vi "Scope_Data.vi"(0 "VDDA":dbl=3.3, 1 "Enum":T6(ring)=enum."I2C_SU_HD_START", 3 "Record Length":i32=2000000, 5 "error in (no error)":errorcluster) -> (12 "output cluster":T1={"Result_Name_Str1"="tSU_Data_ns", "Result_Val1"=864.0093750000001, "Result_Name_Str2"="tHD_Data_ns", "Result_Val2"=1006.8265625, "Result_P/F__Str"="PASSED", "Result_Bool"=TRUE}, 14 "SU_DATA(ns)":dbl=864.0093750000001, 15 "HD_DATA(ns)":dbl=1006.8265625, 16 "ACKs":T3={"Reg Address ACK"=TRUE, "Address ACK"=TRUE, "Data ACK"=TRUE}, 17 "Address_Data":T2={"Data"=82, "Address"=77, "Reg Address"=102} {"Data" format="%.0x"; "Address" format="%.0x"; "Reg Address" format="%.0x"}, 19 "error out":errorcluster)   [LabVIEW 2019]
uses:
  <vilib>/addons/jitter/shared/controls/ja_crossing times.ctl
  <vilib>/addons/jitter/shared/controls/ja_slope (two options).ctl
  <vilib>/addons/jitter/shared/controls/ja_state_settings.ctl
  <vilib>/addons/jitter/shared/controls/ja_reference level settings.ctl
  <userlib>/_TI-LA/Instr Drivers/Oscilloscope/MSO5X/Driver/Base/Public/Data/Low Level/Fetch (Waveform).vi
  <vilib>/addons/jitter/level/support/State Levels (DBL).vi
  <vilib>/addons/jitter/level/support/Reference Levels (waveform in, DBL).vi
  <vilib>/addons/jitter/level/support/Find Transitions (DBL).vi
  <vilib>/addons/jitter/timing/support/Level Crossing (Transitions in, DBL).vi
  <userlib>/_TI-LA/Instr Drivers/Oscilloscope/MSO5X/Driver/Base/Tektronix MSO5X Series.lvlib
  <vilib>/addons/jitter/NI_JAT.lvlib
panel:
  out "tBUF(ns)":dbl=32.37685263084059
  out "Result_Name_Str2":string="tHD_Data_ns"
  out "Result_Name_Str1":string="tSU_Data_ns"
  out "Result_Val2":dbl=1006.8265625 format="%#_13g"
  out "Result_Val1":dbl=864.0093750000001 format="%#_13g"
  out "Result_P/F__Str":string="PASSED"
  out "tHIGH(ns)":dbl=0.9820852205979463
  out "tLOW(ns)":dbl=32.37685263084059
  out "HD_START(ns) 400K":dbl=0.9820852205979463
  out "SU_START(ns) 400K":dbl=32.37685263084059
  out "SU_STOP(ns)":dbl=32.37685263084059
  in  "crossing level 2":dbl=nan
  out "error out 2":errorcluster
  out "level crossings 2":T4={"indexes"=[138886.34765625, 144273.98567708334, 150623.021484375, 168977.31901041666, 175242.021484375, 177621.478515625, 183858.04296875, 194311.65234375, 200551.01432291666, 217971.31901041666, 221517.021484375, 227093.31901041666, 233441.521484375, 251871.978515625, 258263.021484375, 260683.95703125, 266952.021484375, 277424.478515625, 283695.0143229167, 302509.95703125, 308780.521484375, 319308.478515625, 325619.521484375, 343952.978515625, 350295.0143229167, 379433.478515625], "t0"=timestamp(3.199999999681756e-10 s since 1904-01-01), "dt"=3.2e-10, "slope"=-1, "crossing level"=1.5548437499999999} {"crossing level" format="%#_6p"; "slope" items=["Rising Edge"=1, "Falling Edge"=-1]; "dt" format="%#_6p"}
  out "waveform dup 2":waveform(dbl)={"t0"=timestamp(3.199999999681756e-10 s since 1904-01-01), "dt"=3.2e-10, "Y"=array[2000000 elements]}
  out "Clock_size":i32=62
  out "Reg Address  Binary":bool[](array[boolean])=[FALSE, TRUE, TRUE, FALSE, FALSE, TRUE, TRUE]
  out "Reg Address ACK":bool=TRUE
  out "Reg Address":u32=102 format="%.0x"
  out "Address Binary":bool[](array[boolean])=[TRUE, FALSE, TRUE, TRUE, FALSE, FALSE, TRUE]
  out "Address ACK":bool=TRUE
  out "Address":u32=77 format="%.0x"
  out "Data ACK":bool=TRUE
  out "Data":u32=82 format="%.0x"
  out "Data Binary":bool[](array[boolean])=[FALSE, TRUE, FALSE, FALSE, TRUE, FALSE, TRUE, FALSE]
  out "Ch2 Waveform Graph":waveform(dbl)(graph)={"t0"=timestamp(3.199999999681756e-10 s since 1904-01-01), "dt"=3.2e-10, "Y"=array[2000000 elements]}
  in  "Channel (CH2)":string="CH4\nCH4"
  out "waveform dup":waveform(dbl)={"t0"=timestamp(3.199999999681756e-10 s since 1904-01-01), "dt"=3.2e-10, "Y"=array[2000000 elements]}
  out "level crossings":T4={"indexes"=[134617.7548828125, 136769.490234375, 140906.7548828125, 145395.7451171875, 149365.509765625, 153842.7451171875, 157724.509765625, 161770.490234375, 165654.7548828125, 170056.490234375, 173946.2548828125, 178701.490234375, 182599.509765625, 187087.2451171875, 190983.7548828125, 195395.2451171875, 199290.7548828125, 203779.49674479166, 207673.2548828125, 211846.7451171875, 215894.2548828125, 220221.490234375, 223687.7548828125, 228251.7451171875, 232184.509765625, 236707.490234375, 240600.7548828125, 244653.7451171875, 248545.7548828125, 252990.490234375, 256888.509765625, 261725.7451171875, 265615.8365885417, 270174.2451171875, 274060.509765625, 278504.490234375, 282399.509765625, 286883.2451171875, 290775.509765625, 295023.7451171875, 299027.509765625, 303667.490234375, 307560.7548828125, 312007.7451171875, 315943.509765625, 320467.7451171875, 324324.2548828125, 328843.830078125, 332734.7548828125, 336709.490234375, 340632.509765625, 345108.7451171875, 349036.8365885417, 353441.7451171875, 357333.509765625, 361309.830078125, 365239.7548828125, 369413.490234375, 373381.7548828125, 377436.490234375, 381484.2548828125, 383687.7451171875], "t0"=timestamp(3.199999999681756e-10 s since 1904-01-01), "dt"=3.2e-10, "slope"=-1, "crossing level"=1.7388281250000002} {"crossing level" format="%#_6p"; "slope" items=["Rising Edge"=1, "Falling Edge"=-1]; "dt" format="%#_6p"}
  in  "crossing level":dbl=nan
  out "VISA resource name out":refnum<visa-resource-name>="MSO54_D03"
  out "Ch1 Waveform Graph":waveform(dbl)(graph)={"t0"=timestamp(3.199999999681756e-10 s since 1904-01-01), "dt"=3.2e-10, "Y"=array[2000000 elements]}
  in  "VISA resource name":refnum<visa-resource-name>="MSO54_D03"
  in  "Channel (CH1)":string="CH1"
  in  "Maximum Time (100000ms)":u32=100000
  in  "Starting Point (1)":i32=1
  in  "Ref Waveform Type":u16(ring) items=["Normal", "Came from a MATH"]
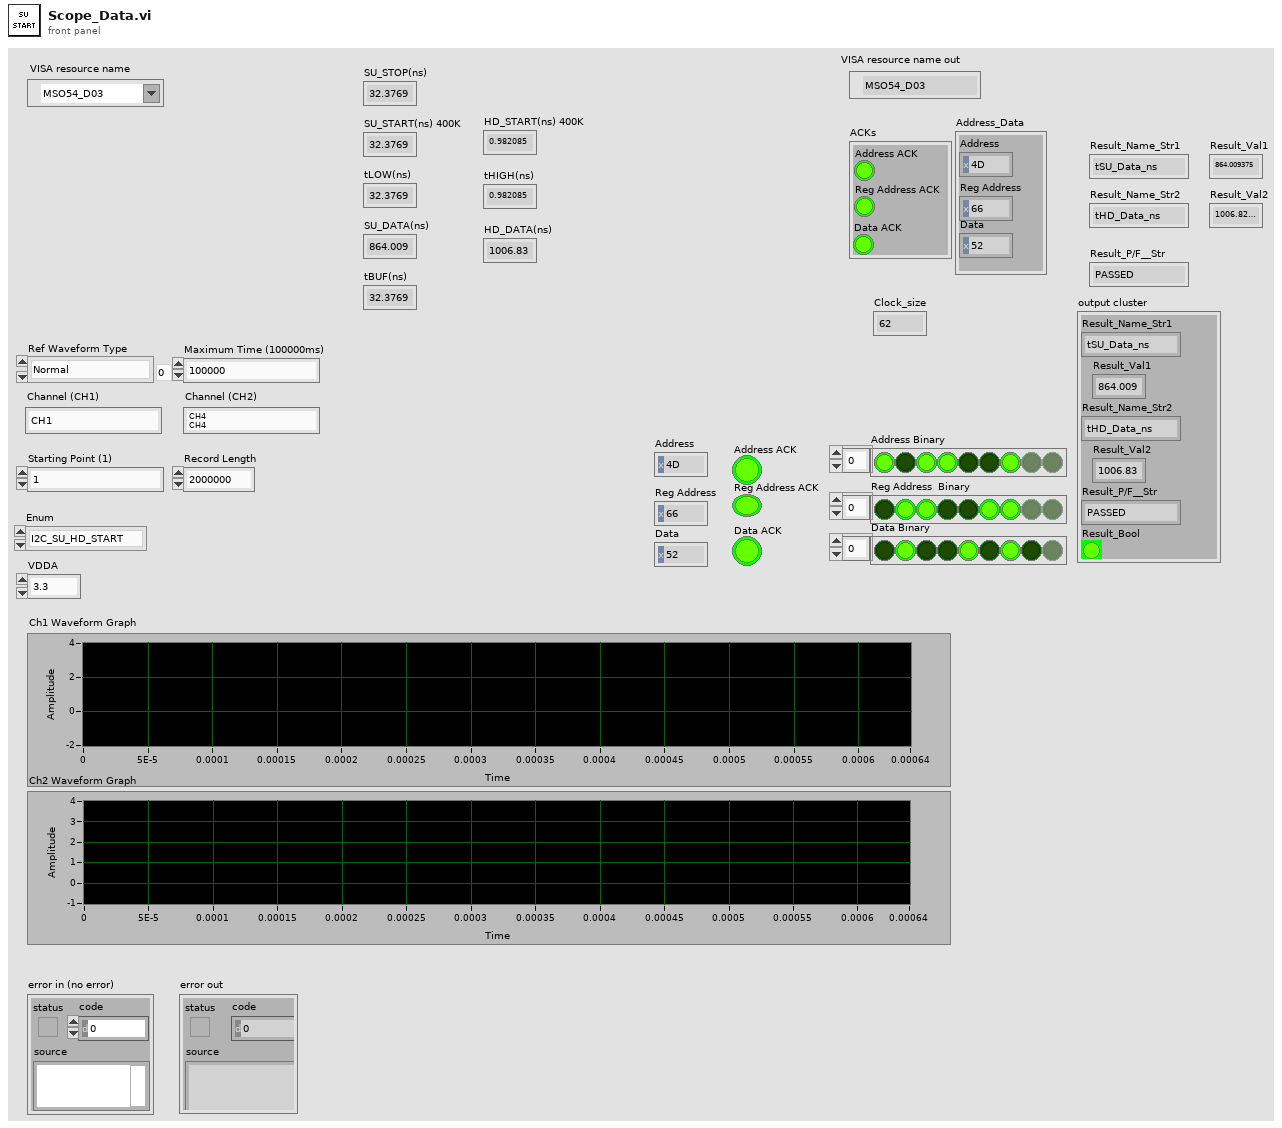
[diagram p1: front panel]
types:
  T1 = cluster{"Result_Name_Str1":string, "Result_Val1":dbl, "Result_Name_Str2":string, "Result_Val2":dbl, "Result_P/F__Str":string, "Result_Bool":bool}
  T2 = cluster{"Data":u32, "Address":u32, "Reg Address":i8}
  T3 = cluster{"Reg Address ACK":bool, "Address ACK":bool, "Data ACK":bool}
  T4 = typedef "NI_JAT.lvlib/ja_crossing times.ctl" = cluster{"indexes":dbl[], "t0":timestamp, "dt":dbl, "slope":T5, "crossing level":dbl}
  T5 = typedef "NI_JAT.lvlib/ja_slope (two options).ctl" = i16
  T6 = enum16{"I2C_Single_byte", "I2C_SU_HD_START", "I2C_SU_HD_DATA", "I2C_SU_STOP", "I2C_CLOCK_HIGH_LOW", "I2C_BUF"}
  T7 = cluster{"Data":u32, "Address":u32, "Reg Address":u32}
  T8 = typedef "NI_JAT.lvlib/ja_state_settings.ctl" = cluster{"method":enum32{"histogram", "peak", "auto select", "auto select independent"}, "histogram size":i32, "histogram method":enum16{"mode"}, "search width/total bins":dbl}
  T9 = typedef "NI_JAT.lvlib/ja_reference level settings.ctl" = cluster{"high ref level":dbl, "mid ref level":dbl, "low ref level":dbl, "ref units":u16}
  T10 = typedef "NI_JAT.lvlib/ja_state_levels.ctl" = cluster{"amplitude":dbl, "high state level":dbl, "low state level":dbl}
  T11 = typedef "NI_JAT.lvlib/ja_reference level.ctl" = cluster{"high ref level":dbl, "mid ref level":dbl, "low ref level":dbl}
  T12 = typedef "NI_JAT.lvlib/ja_transition.ctl" = cluster{"transition":T13[], "state levels":T10, "ref levels":T11}
  T13 = typedef "NI_JAT.lvlib/ja_edge.ctl" = cluster{"start index":dbl, "end index":dbl, "slope":T5}
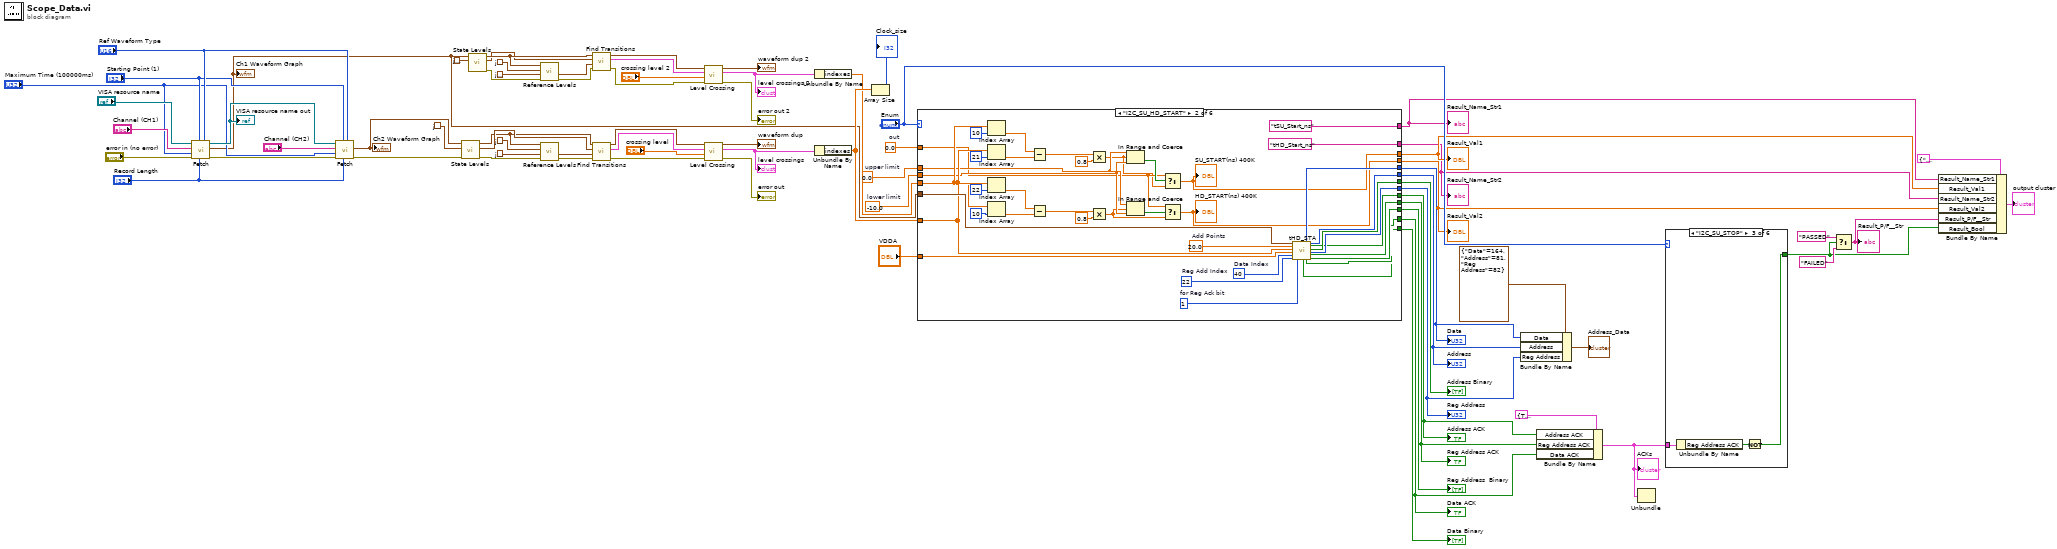
[diagram p0: block diagram]
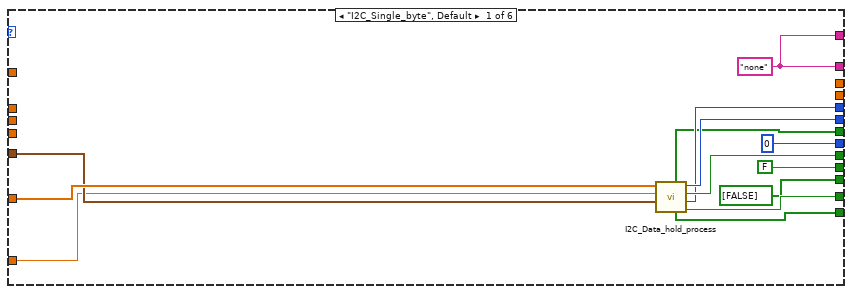
[diagram p2: hidden frame]
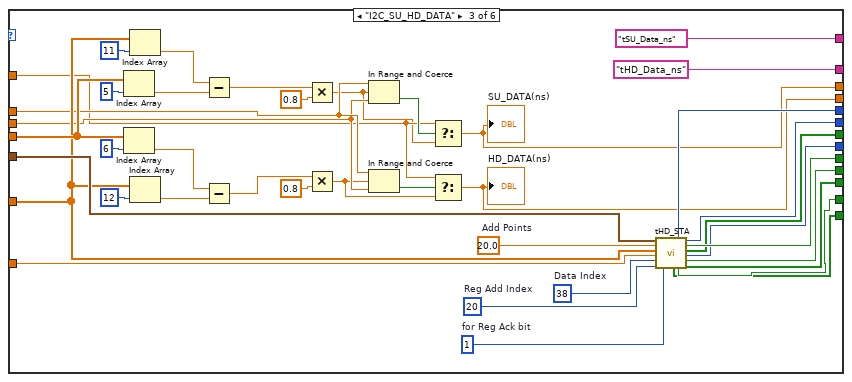
[diagram p3: hidden frame]
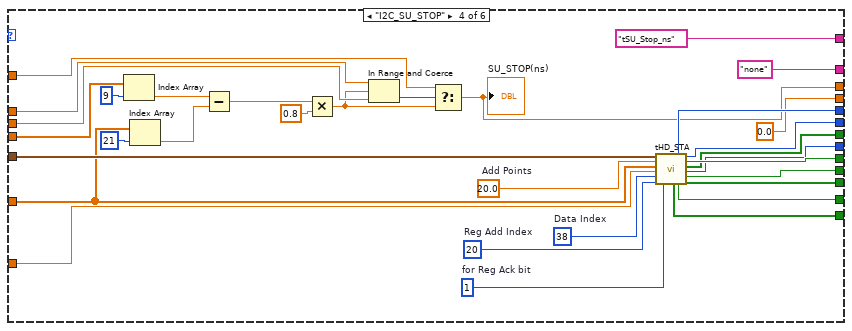
[diagram p4: hidden frame]
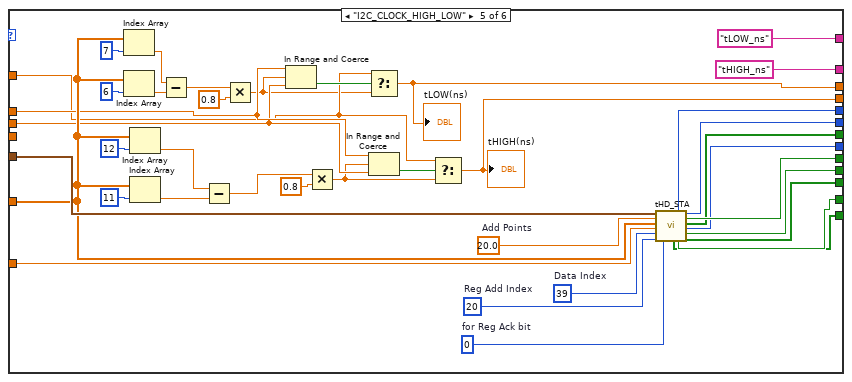
[diagram p5: hidden frame]
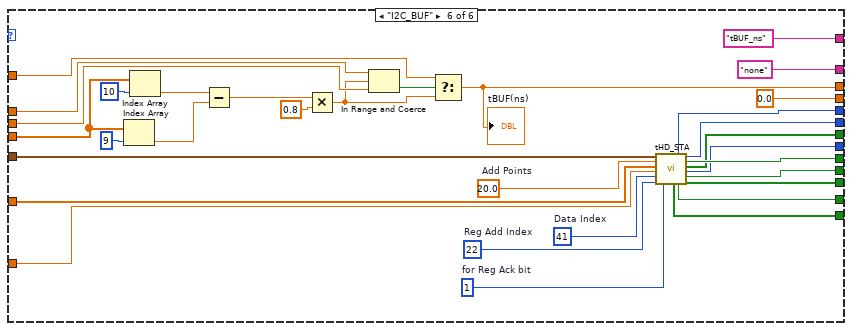
[diagram p6: hidden frame]
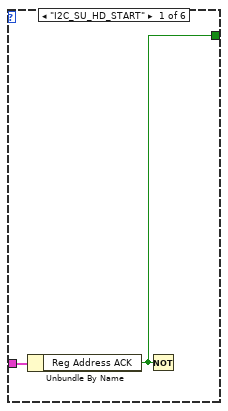
[diagram p7: hidden frame]
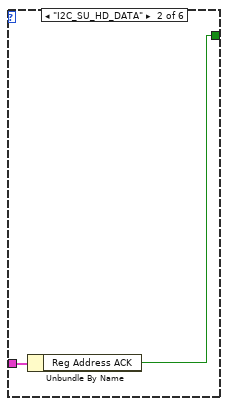
[diagram p8: hidden frame]
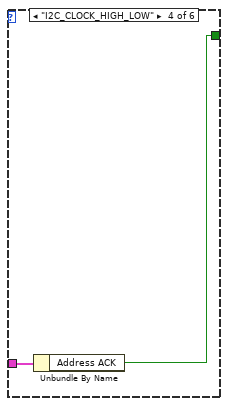
[diagram p9: hidden frame]
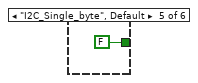
[diagram p10: hidden frame]
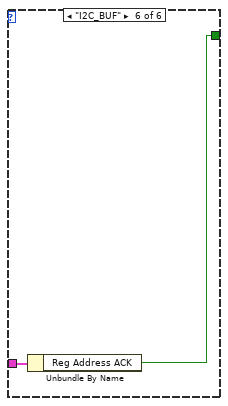
[diagram p11: hidden frame]
diagram:
  w14 = 0.0  # out
  w15 = -10.0  # lower limit
  w16 = 0.0  # upper limit
  n1 = call-poly <userlib>:"Fetch.vi"("Ref Waveform Type"="Ref Waveform Type", "Ending Point (2500)"="Record Length", "Starting Point (1)"="Starting Point (1)", "error in (no error)"="error in (no error)", "Maximum Time (100000ms)"="Maximum Time (100000ms)", "Channel (CH1)"="Channel (CH1)", "VISA resource name"="VISA resource name") -> ("error out"=w57:errorcluster, "Waveform Graph"=w29:waveform(dbl), "VISA resource name out"=w56:refnum<visa-resource-name>)  [unwired: 2 in]
  "Ch1 Waveform Graph" <- w29
  "VISA resource name out" <- w56
  n2 = call-poly <userlib>:"Fetch.vi"("Ref Waveform Type"="Ref Waveform Type", "Ending Point (2500)"="Record Length", "Starting Point (1)"="Starting Point (1)", "error in (no error)"=w57, "Maximum Time (100000ms)"="Maximum Time (100000ms)", "Channel (CH1)"="Channel (CH2)", "VISA resource name"=w56) -> ("error out"=w51:errorcluster, "Waveform Graph"=w52:waveform(dbl))  [unwired: 2 in, 1 out]
  "Ch2 Waveform Graph" <- w52
  n3 = call-poly <vilib>:"State Levels.vi"("error in"=w51, "state levels settings"=T8 {"method"=enum."histogram", "histogram size"=256, "histogram method"=enum."mode", "search width/total bins"=0.45}, "waveform"=w52) -> ("error out"=w49:errorcluster, "state levels"=w68:T10, "waveform dup"=w64:waveform(dbl))  [unwired: 6 in]
  n4 = call-poly <vilib>:"State Levels.vi"("state levels settings"=T8 {"method"=enum."histogram", "histogram size"=256, "histogram method"=enum."mode", "search width/total bins"=0.45}, "waveform"=w29) -> ("error out"=w43:errorcluster, "state levels"=w33:T10, "waveform dup"=w37:waveform(dbl))  [unwired: 7 in]
  n5 = call-poly <vilib>:"Reference Levels.vi"("error in"=w43, "reference levels settings"=T9 {"high ref level"=90.0, "mid ref level"=50.0, "low ref level"=10.0, "ref units"=1}, "state levels settings"=T8 {"method"=enum."histogram", "histogram size"=256, "histogram method"=enum."mode", "search width/total bins"=0.45} ("state levels settings 2"), "waveform"=w37) -> ("error out"=w44:errorcluster, "reference levels"=w40:T11)  [unwired: 4 in, 2 out]
  n6 = call-poly <vilib>:"Reference Levels.vi"("error in"=w49, "reference levels settings"=T9 {"high ref level"=90.0, "mid ref level"=50.0, "low ref level"=10.0, "ref units"=1}, "state levels settings"=T8 {"method"=enum."histogram", "histogram size"=256, "histogram method"=enum."mode", "search width/total bins"=0.45} ("state levels settings 2"), "waveform"=w64) -> ("error out"=w48:errorcluster, "reference levels"=w61:T11)  [unwired: 4 in, 2 out]
  n7 = call-poly <vilib>:"Find Transitions.vi"("error in (no error)"=w44, "reference levels"=w40, "state levels"=w33, "waveform"=w37) -> ("error out"=w42:errorcluster, "transitions"=w35:T12, "waveform dup"=w34:waveform(dbl))  [unwired: 5 in]
  n8 = call-poly <vilib>:"Find Transitions.vi"("error in (no error)"=w48, "reference levels"=w61, "state levels"=w68, "waveform"=w64) -> ("error out"=w50:errorcluster, "transitions"=w66:T12, "waveform dup"=w67:waveform(dbl))  [unwired: 5 in]
  n9 = call-poly <vilib>:"Level Crossing.vi"("error in (no error)"=w42, "crossing level"="crossing level 2", "transitions"=w35, "waveform"=w34) -> ("error out"=→"error out 2":errorcluster, "level crossings"=w41:T4, "waveform dup"=→"waveform dup 2":waveform(dbl))  [unwired: 5 in]
  "level crossings 2" <- w41
  n10 = call-poly <vilib>:"Level Crossing.vi"("error in (no error)"=w50, "crossing level"="crossing level", "transitions"=w66, "waveform"=w67) -> ("error out"=→"error out":errorcluster, "level crossings"=w60:T4, "waveform dup"=→"waveform dup":waveform(dbl))  [unwired: 5 in]
  "level crossings" <- w60
  n11 = Unbundle By Name(w41) -> ("indexes"=w28:dbl[])
  n12 = Unbundle By Name(w60) -> ("indexes"=w46:dbl[])
  n13 = Array Size(array=w46) -> (size(s)=→"Clock_size":i32)
  n14 = case shown="\"I2C_SU_HD_START\"" "Enum" {
    tunnel: w46 -> [w87 w108 w146 w181 w219 w263]
    tunnel: w29 -> [w86 w126 w167 w199 w238 w264]
    tunnel: "VDDA" -> [w85 w127 w166 w198 w237 w239]
    tunnel: [bool[] [FALSE] ("Reg Address  Binary") w125 w159 w189 w230 w254] -> w13
    tunnel: [FALSE ("Reg Address ACK") w124 w160 w190 w231 w255] -> w12
    tunnel: [u32 0 ("Reg Address") w123 w161 w191 w232 w257] -> w11
    tunnel: [w80 w122 w162 w192 w233 w256] -> w10
    tunnel: [w84 w121 w163 w193 w234 w258] -> w9
    tunnel: [w83 w120 w164 w194 w235 w259] -> w8
    tunnel: [w81 w119 w158 w188 w229 w253] -> w7
    tunnel: [w82 w118 w165 w195 w236 w260] -> w6
    tunnel: [w79 w117 w157 w187 w228 w252] -> w5
    tunnel: w28 -> [_ w107 w148 w182 _ w251]
    tunnel: [w75 "tSU_Start_ns" "tSU_Data_ns" "tSU_Stop_ns" "tLOW_ns" "tBUF_ns"] -> w4
    tunnel: [_ w100 w139 w175 w212 w249] -> w3
    tunnel: [w75 "tHD_Start_ns" "tHD_Data_ns" "none" "tHIGH_ns" "none"] -> w2
    tunnel: [_ w99 w140 0.0 w211 0.0] -> w1
    tunnel: w16 -> [_ w96 w136 w173 w208 w247]
    tunnel: w15 -> [_ w95 w135 w172 w207 w246]
    tunnel: w14 -> [_ w94 w134 w171 w206 w245]
    frame "I2C_Single_byte", Default {
      w75 = "none"
      n15 = call "I2C_Data_hold_process.vi"("waveform"=w86, "VDDA"=w85, "Index"=w87) -> ("Data ACK"=w81:bool, "Data"=w82:u32, "Address ACK"=w84:bool, "Address"=w83:u32, "Data Binary"=w79:bool[], "Address Binary"=w80:bool[])  [unwired: 3 in]
    }
    frame "I2C_SU_HD_START" {
      w89 = 1  # for Reg Ack bit
      w88 = 20.0  # Add Points
      w91 = 22  # Reg Add Index
      w90 = 40  # Data Index
      n16 = Index Array(array=w107, index=10) -> (element=w105:dbl)
      n17 = Index Array(array=w108, index=21) -> (element=w106:dbl)
      n18 = Index Array(array=w108, index=22) -> (element=w103:dbl)
      n19 = Index Array(array=w107, index=10) -> (element=w104:dbl)
      n20 = Subtract(x=w105, y=w106) -> (x-y=w114:dbl)
      n21 = Subtract(x=w103, y=w104) -> (x-y=w110:dbl)
      n22 = Multiply(x=w114, y=0.8) -> (x*y=w93:dbl)
      n23 = Multiply(x=w110, y=0.8) -> (x*y=w92:dbl)
      n24 = In Range and Coerce(upper limit=w96, x=w93, lower limit=w95) -> (In Range?=w98:bool)  [unwired: 1 out]
      n25 = In Range and Coerce(upper limit=w96, x=w92, lower limit=w95) -> (In Range?=w97:bool)  [unwired: 1 out]
      n26 = Select(t=w94, s=w98, f=w93) -> (s? t:f=w100:dbl)
      "SU_START(ns) 400K" <- w100
      n27 = Select(t=w94, s=w97, f=w92) -> (s? t:f=w99:dbl)
      "HD_START(ns) 400K" <- w99
      n28 = call "tHD_STA.vi"("waveform"=w126, "Add Points"=w88, "Index"=w108, "VDDA"=w127, "index 2"=w90, "index"=w91, "for Reg Ack bit"=w89) -> ("Data Binary"=w117:bool[], "Data"=w118:u32, "Data ACK"=w119:bool, "Address"=w120:u32, "Address ACK"=w121:bool, "Address Binary"=w122:bool[], "Reg Address"=w123:u32, "Reg Address ACK"=w124:bool, "Reg Address  Binary"=w125:bool[])  [unwired: 4 in]
    }
    frame "I2C_SU_HD_DATA" {
      w129 = 1  # for Reg Ack bit
      w128 = 20.0  # Add Points
      w130 = 20  # Reg Add Index
      w131 = 38  # Data Index
      n29 = Index Array(array=w148, index=5) -> (element=w153:dbl)
      n30 = Index Array(array=w148, index=6) -> (element=w150:dbl)
      n31 = Index Array(array=w146, index=11) -> (element=w154:dbl)
      n32 = Index Array(array=w146, index=12) -> (element=w149:dbl)
      n33 = Subtract(x=w154, y=w153) -> (x-y=w152:dbl)
      n34 = Subtract(x=w150, y=w149) -> (x-y=w144:dbl)
      n35 = Multiply(x=w152, y=0.8) -> (x*y=w132:dbl)
      n36 = Multiply(x=w144, y=0.8) -> (x*y=w133:dbl)
      n37 = In Range and Coerce(upper limit=w136, x=w132, lower limit=w135) -> (In Range?=w138:bool)  [unwired: 1 out]
      n38 = In Range and Coerce(upper limit=w136, x=w133, lower limit=w135) -> (In Range?=w137:bool)  [unwired: 1 out]
      n39 = Select(t=w134, s=w138, f=w132) -> (s? t:f=w139:dbl)
      "SU_DATA(ns)" <- w139
      n40 = Select(t=w134, s=w137, f=w133) -> (s? t:f=w140:dbl)
      "HD_DATA(ns)" <- w140
      n41 = call "tHD_STA.vi"("waveform"=w167, "Add Points"=w128, "Index"=w146, "VDDA"=w166, "index 2"=w131, "index"=w130, "for Reg Ack bit"=w129) -> ("Data Binary"=w157:bool[], "Data"=w165:u32, "Data ACK"=w158:bool, "Address"=w164:u32, "Address ACK"=w163:bool, "Address Binary"=w162:bool[], "Reg Address"=w161:u32, "Reg Address ACK"=w160:bool, "Reg Address  Binary"=w159:bool[])  [unwired: 4 in]
    }
    frame "I2C_SU_STOP" {
      w168 = 1  # for Reg Ack bit
      w169 = 20.0  # Add Points
      w196 = 20  # Reg Add Index
      w197 = 38  # Data Index
      n42 = Index Array(array=w182, index=9) -> (element=w180:dbl)
      n43 = Index Array(array=w181, index=21) -> (element=w179:dbl)
      n44 = Subtract(x=w180, y=w179) -> (x-y=w184:dbl)
      n45 = Multiply(x=w184, y=0.8) -> (x*y=w170:dbl)
      n46 = In Range and Coerce(upper limit=w173, x=w170, lower limit=w172) -> (In Range?=w174:bool)  [unwired: 1 out]
      n47 = Select(t=w171, s=w174, f=w170) -> (s? t:f=w175:dbl)
      "SU_STOP(ns)" <- w175
      n48 = call "tHD_STA.vi"("waveform"=w199, "Add Points"=w169, "Index"=w181, "VDDA"=w198, "index 2"=w197, "index"=w196, "for Reg Ack bit"=w168) -> ("Data Binary"=w187:bool[], "Data"=w195:u32, "Data ACK"=w188:bool, "Address"=w194:u32, "Address ACK"=w193:bool, "Address Binary"=w192:bool[], "Reg Address"=w191:u32, "Reg Address ACK"=w190:bool, "Reg Address  Binary"=w189:bool[])  [unwired: 4 in]
    }
    frame "I2C_CLOCK_HIGH_LOW" {
      w201 = 0  # for Reg Ack bit
      w200 = 20.0  # Add Points
      w202 = 20  # Reg Add Index
      w203 = 39  # Data Index
      n49 = Index Array(array=w219, index=7) -> (element=w218:dbl)
      n50 = Index Array(array=w219, index=6) -> (element=w217:dbl)
      n51 = Index Array(array=w219, index=12) -> (element=w216:dbl)
      n52 = Index Array(array=w219, index=11) -> (element=w215:dbl)
      n53 = Subtract(x=w218, y=w217) -> (x-y=w225:dbl)
      n54 = Subtract(x=w216, y=w215) -> (x-y=w221:dbl)
      n55 = Multiply(x=w225, y=0.8) -> (x*y=w205:dbl)
      n56 = In Range and Coerce(upper limit=w208, x=w205, lower limit=w207) -> (In Range?=w209:bool)  [unwired: 1 out]
      n57 = Multiply(x=w221, y=0.8) -> (x*y=w204:dbl)
      n58 = Select(t=w206, s=w209, f=w205) -> (s? t:f=w212:dbl)
      "tLOW(ns)" <- w212
      n59 = In Range and Coerce(upper limit=w208, x=w204, lower limit=w207) -> (In Range?=w210:bool)  [unwired: 1 out]
      n60 = Select(t=w206, s=w210, f=w204) -> (s? t:f=w211:dbl)
      "tHIGH(ns)" <- w211
      n61 = call "tHD_STA.vi"("waveform"=w238, "Add Points"=w200, "Index"=w219, "VDDA"=w237, "index 2"=w203, "index"=w202, "for Reg Ack bit"=w201) -> ("Data Binary"=w228:bool[], "Data"=w236:u32, "Data ACK"=w229:bool, "Address"=w235:u32, "Address ACK"=w234:bool, "Address Binary"=w233:bool[], "Reg Address"=w232:u32, "Reg Address ACK"=w231:bool, "Reg Address  Binary"=w230:bool[])  [unwired: 4 in]
    }
    frame "I2C_BUF" {
      w241 = 1  # for Reg Ack bit
      w240 = 20.0  # Add Points
      w243 = 22  # Reg Add Index
      w242 = 41  # Data Index
      n62 = Index Array(array=w251, index=9) -> (element=w266:dbl)
      n63 = Index Array(array=w251, index=10) -> (element=w265:dbl)
      n64 = Subtract(x=w265, y=w266) -> (x-y=w269:dbl)
      n65 = Multiply(x=w269, y=0.8) -> (x*y=w244:dbl)
      n66 = In Range and Coerce(upper limit=w247, x=w244, lower limit=w246) -> (In Range?=w248:bool)  [unwired: 1 out]
      n67 = Select(t=w245, s=w248, f=w244) -> (s? t:f=w249:dbl)
      "tBUF(ns)" <- w249
      n68 = call "tHD_STA.vi"("waveform"=w264, "Add Points"=w240, "Index"=w263, "VDDA"=w239, "index 2"=w242, "index"=w243, "for Reg Ack bit"=w241) -> ("Data Binary"=w252:bool[], "Data"=w260:u32, "Data ACK"=w253:bool, "Address"=w259:u32, "Address ACK"=w258:bool, "Address Binary"=w256:bool[], "Reg Address"=w257:u32, "Reg Address ACK"=w255:bool, "Reg Address  Binary"=w254:bool[])  [unwired: 4 in]
    }
  }
  "Data Binary" <- w5
  "Data" <- w6
  "Data ACK" <- w7
  "Address" <- w8
  "Address ACK" <- w9
  "Address Binary" <- w10
  "Reg Address" <- w11
  "Reg Address ACK" <- w12
  "Reg Address  Binary" <- w13
  "Result_Val1" <- w3
  "Result_Val2" <- w1
  "Result_Name_Str1" <- w4
  "Result_Name_Str2" <- w2
  n69 = Bundle By Name(cluster=T7 {"Data"=164, "Address"=81, "Reg Address"=82}, "Data"=w6, "Address"=w8, "Reg Address"=w11) -> (→"Address_Data":T7)
  n70 = Bundle By Name(cluster=T3 {"Reg Address ACK"=TRUE, "Address ACK"=TRUE, "Data ACK"=TRUE}, "Address ACK"=w9, "Reg Address ACK"=w12, "Data ACK"=w7) -> (w23:T3)
  "ACKs" <- w23
  n71 = Unbundle(w23) -> ()  [unwired: 3 out]
  n72 = case shown="\"I2C_SU_STOP\"" "Enum" {
    tunnel: w23 -> [w272 w274 w277 w279 _ w282]
    tunnel: [w271 w273 w275 w278 FALSE ("Address ACK") w281] -> w18
    frame "I2C_SU_HD_START" {
      n73 = Unbundle By Name(w272) -> ("Reg Address ACK"=w271:bool)
      n74 = Not(x=w271) -> ()  [unwired: 1 out]
    }
    frame "I2C_SU_HD_DATA" {
      n75 = Unbundle By Name(w274) -> ("Reg Address ACK"=w273:bool)
    }
    frame "I2C_SU_STOP" {
      n76 = Unbundle By Name(w277) -> ("Reg Address ACK"=w276:bool)
      n77 = Not(x=w276) -> (.not. x?=w275:bool)
    }
    frame "I2C_CLOCK_HIGH_LOW" {
      n78 = Unbundle By Name(w279) -> ("Address ACK"=w278:bool)
    }
    frame "I2C_Single_byte", Default {
    }
    frame "I2C_BUF" {
      n79 = Unbundle By Name(w282) -> ("Reg Address ACK"=w281:bool)
    }
  }
  n80 = Select(t="PASSED", s=w18, f="FAILED") -> (s? t:f=w19:string)
  "Result_P/F__Str" <- w19
  n81 = Bundle By Name(cluster=T1 {"Result_Name_Str1"="tLOW_ns", "Result_Val1"=469.0, "Result_Name_Str2"="tHIGH_ns", "Result_Val2"=29.0, "Result_P/F__Str"="PASSED", "Result_Bool"=TRUE}, "Result_Name_Str1"=w4, "Result_Val1"=w3, "Result_Name_Str2"=w2, "Result_Val2"=w1, "Result_P/F__Str"=w19, "Result_Bool"=w18) -> (→"output cluster":T1)
